vi "CC Swap Script Steps.vi"(8 "error in (no error)":errorcluster, 10 "index":i32, 11 "Script in":T1[](array[typedef])) -> (0 "error out":errorcluster, 3 "Script out":T1[](array[typedef]))   [LabVIEW 2021]
uses:
  typedefs/CC Script Step.ctl
  typedefs/CC enum Script Action.ctl
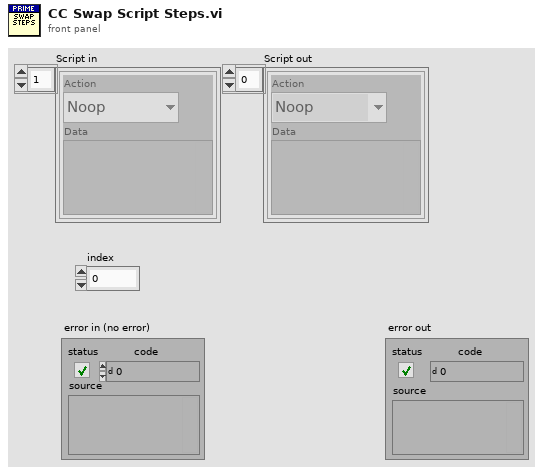
[diagram p1: front panel]
types:
  T1 = typedef "CC Script Step.ctl" = cluster{"Action":T2, "Data":variant}
  T2 = typedef "CC enum Script Action.ctl" = enum16{"Noop", "Define Object", "Define Exposure", "Define Dithering", "Acquire Images", "Set Filter Wheel", "Telescope Home", "Telescope Move", "Telescope RA DEC", "Focus Move Relative", "Focus Move Absolute", "Focus Set Home", "Macro", "Pause", "Ask User", "Define Random Dither"}
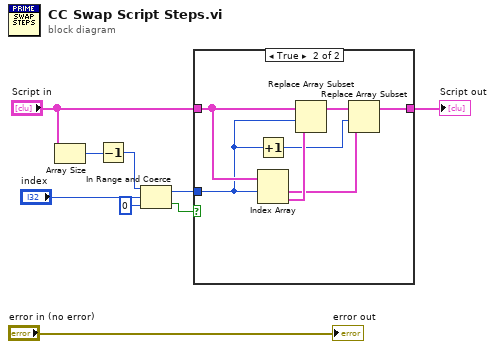
[diagram p0: block diagram]
diagram:
  n1 = Array Size(array="Script in") -> (size(s)=w7:i32)
  n2 = Decrement(x=w7) -> (x-1=w1:i32)
  n3 = In Range and Coerce(upper limit=w1, x="index", lower limit=0) -> (coerced(x)=w4:i32, In Range?=w3:bool)
  n4 = case shown="True" w3 {
    tunnel: "Script in" -> [w10 w13]
    tunnel: w4 -> [_ w12]
    tunnel: [w10 w14] -> w2
    frame False {
    }
    frame True {
      n5 = Increment(x=w12) -> (x+1=w11:i32)
      n6 = Index Array(array=w13, index #1=w12) -> (element #1=w16:T1, element #2=w17:T1)  [unwired: 1 in]
      n7 = Replace Array Subset(array=w13, new element=w17, index=w12) -> (w15:T1[])
      n8 = Replace Array Subset(array=w15, new element=w16, index=w11) -> (w14:T1[])
    }
  }
  "Script out" <- w2
  "error out" <- "error in (no error)"
